vi "FPGA_main_AIchar_v3.vi"() -> ()   [LabVIEW 2020]
doc: "AI from AI modules, Mod6, Mod7, Mod8"
uses:
  <vilib>/rvi/Emulation/niFpgaGetClockAttributes.vi
  <vilib>/rvi/Emulation/niFpgaSctlEmulationGetInTimedLoop.vi
  <vilib>/rvi/Emulation/niFpgaEmulationReportErrorSimple.vi
  <vilib>/rvi/eio/common/nirviEmuTemplateMethod_errors.vi
  <vilib>/rvi/Emulation/niFpgaEmulationIsFPGAContextNoSignature.vi
  <vilib>/rvi/errors/niFpgaSetErrorForExecOnDevCompSimple.vi
  <vilib>/rvi/eio/common/nirviEmuReportErrorAndStop.vi
  <vilib>/rvi/DataTransferAndStorage/Container/Common/niFpgaContainerGetUniqueNameForEmu.vi
  <vilib>/rvi/FIFO/Fifo_Resource/nirvififoEmulationSetSize.vi
  <vilib>/rvi/FIFO/Fifo_Resource/nirviFifoEmulationQueueMgr.vi
  <instcachedir>/0/nirviFifoEmulationQueueMgr_E5CAEC123FF24DC58D834DCA3CDAA9B5.lvgen/nirviFifoEmulationQueueMgr_E5CAEC123FF24DC58D834DCA3CDAA9B5_001.vi
  <vilib>/rvi/FIFO/Fifo_Resource/nirvififoEmulationDetermineInputValidOut.vi
  <vilib>/rvi/FIFO/Fifo_Resource/nirvififoEmulationCreateLock.vi
  <vilib>/rvi/Emulation/niFpgaProcessEmulError.vi
  <vilib>/rvi/FIFO/Fifo_Resource/nirvififoEmulationObtainLock.vi
  <vilib>/rvi/FIFO/Fifo_Resource/nirvififoEmulationReleaseLock.vi
  <vilib>/rvi/occurrence/nirviWaitOnOccurrenceBase.vi
  <vilib>/rvi/errors/nirviReportUnexpectedCaseInternalError.vi
  <vilib>/rvi/errors/nirviReportUnexpectedCaseInternalError (U32).vi
  <vilib>/rvi/Emulation/niFpgaCriticalErrorInLSC.vi
  <vilib>/Utility/error.llb/Clear Errors.vi
  Components/PositionMeas/MovingAverage/256ptMovingAvg.vi
  Components/PositionMeas/MovingAverage/64ptMovingAvg.vi
  <vilib>/rvi/DataTransferAndStorage/Container/Common/niFpgaContainerSetEmuInfo.vi
  <vilib>/eio/EIONode/EIONode.xnode
  <vilib>/rvi/DataTransferAndStorage/Container/XNode/niFpgaContainer.xnode
  <vilib>/rvi/FIFO/Fifo_Resource/nirvififoEmulationWrite.vi
  <vilib>/rvi/FIFO/Fifo_Resource/nirvififoEmulationRead.vi
  <vilib>/rvi/LocalResourceManager/LocalResourceManager.xnode
  Components/PositionMeas/MovingAverage/MovingAvg.lvlib
panel:
  out "AI LS Loop time [us] 2":u8
  out "FPGA AI LS FIFO\nOverflow? 2":bool
  out "AI LS filter Loop time [us] 2":u8
  out "Mod6 (NI 9222) AI":fxp<+/-,25,5>[](array[numeric])
  out "AI LS filter Loop time [us]":u8
  out "Mod7 (NI 9222) AI":fxp<+/-,25,5>[](array[numeric])
  out "AI LS Loop time [us]":u8
  out "FPGA AI LS FIFO\nOverflow?":bool
  out "Mod8 (NI 9222) AI":fxp<+/-,25,5>[](array[numeric])
  out "AI HS filter Loop time [ticks]":u8
  out "FPGA AI HS FIFO\nOverflow?":bool
  out "AI HS Loop time [ticks]":u8
  # "1 tick = 25 ns"
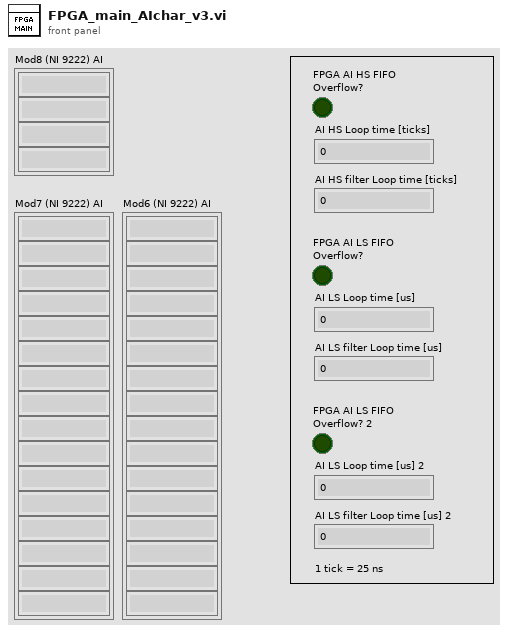
[diagram p1: front panel]
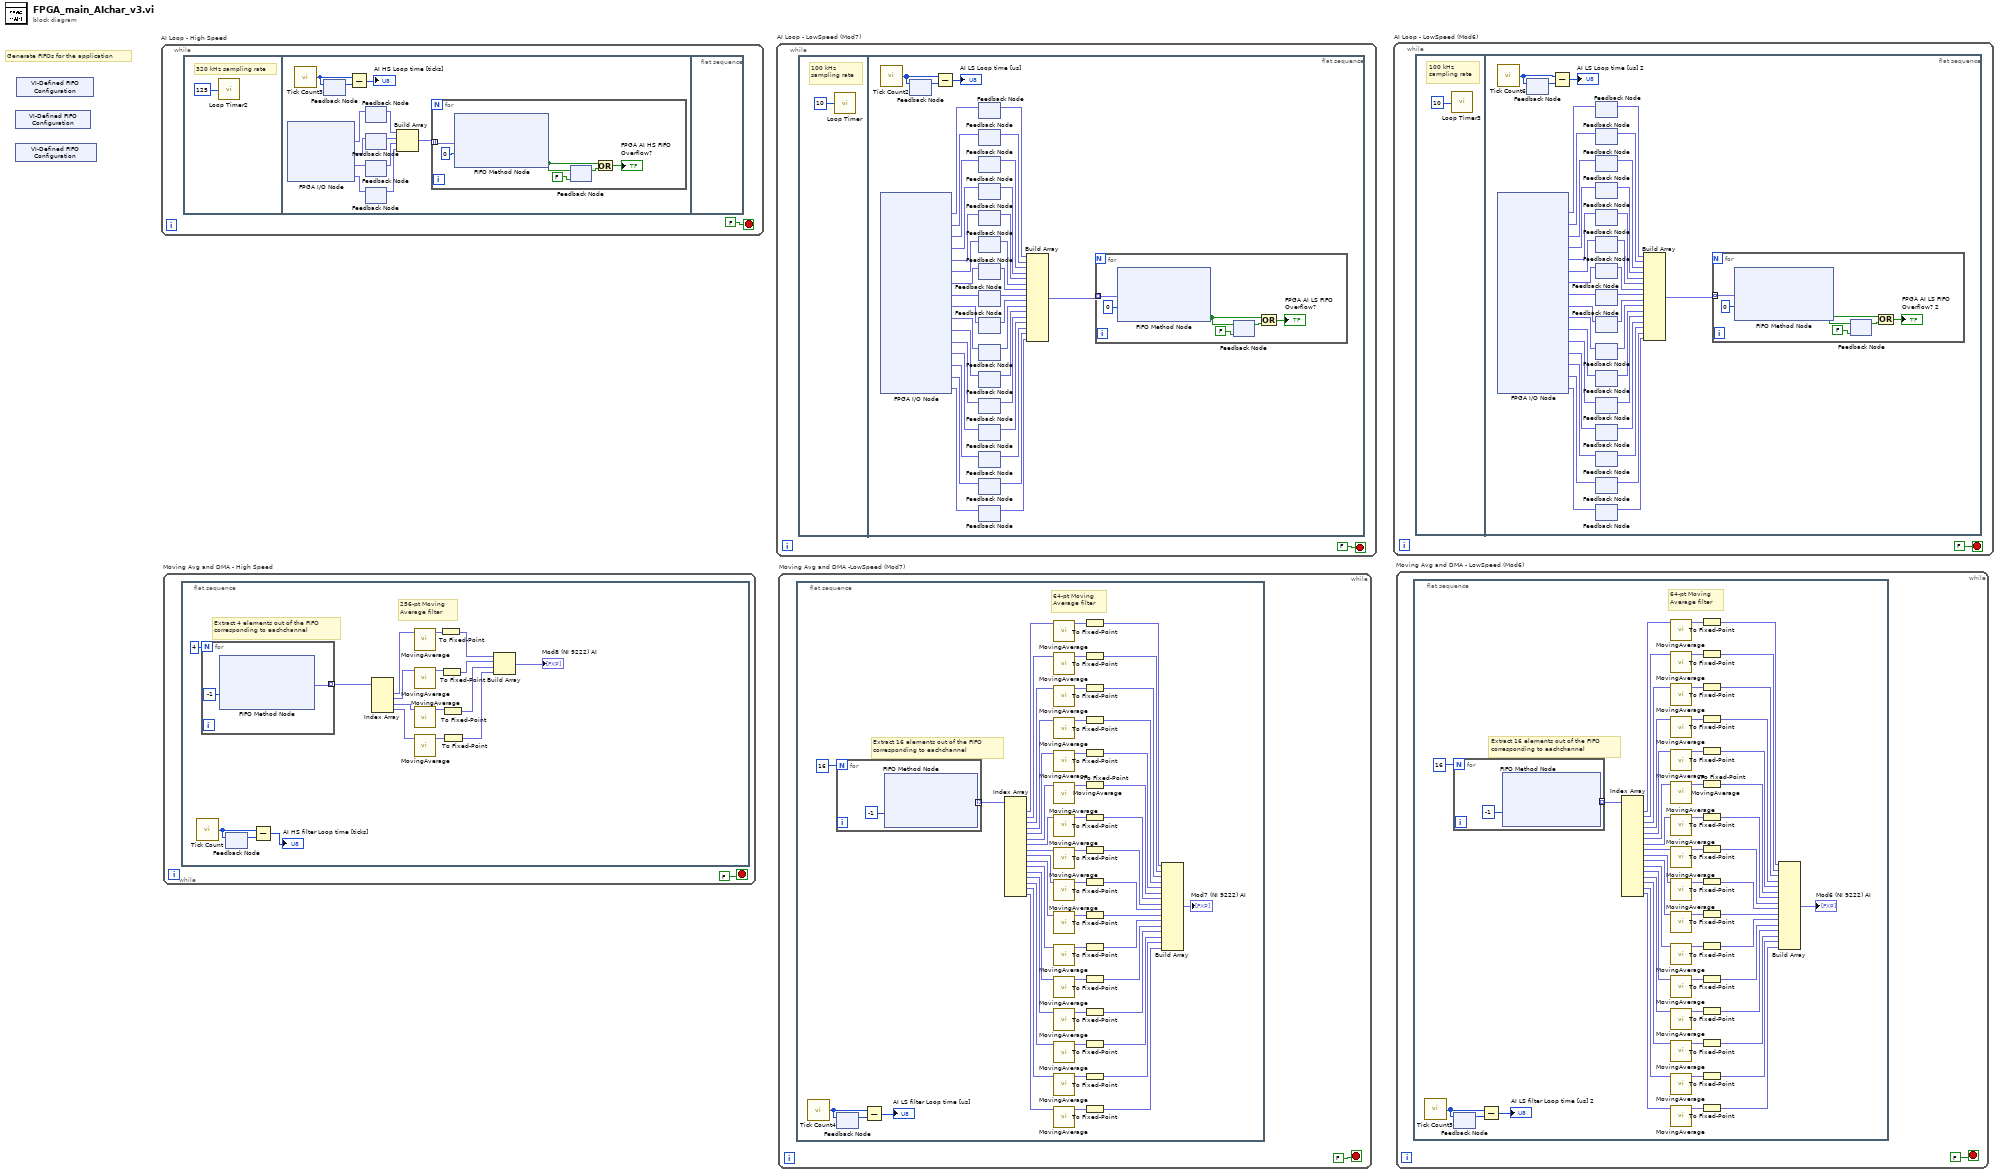
[diagram p0: block diagram]
diagram:
  # "Generate FIFOs for the application"
  n1 = xnode "VI-Defined FIFO Configuration"() -> ()  [unwired: 1 out]
  n2 = xnode "VI-Defined FIFO Configuration"() -> ()  [unwired: 1 out]
  n3 = xnode "VI-Defined FIFO Configuration"() -> ()  [unwired: 1 out]
  n4 = while "AI Loop - High Speed" {
    stop <- FALSE stop-if-true
    n5 = flat-sequence {
      frame #0 {
        # "320 kHz sampling rate"
        n6 = call "Loop Timer2"("Count(Ticks)"=u8 125) -> ()  [unwired: 1 out]
      }
      frame #1 {
        n7 = xnode "FPGA I/O Node"() -> ("Mod8/AI0"=w9:fxp<+/-,24,5>, "Mod8/AI1"=w8:fxp<+/-,24,5>, "Mod8/AI2"=w7:fxp<+/-,24,5>, "Mod8/AI3"=w6:fxp<+/-,24,5>)  [unwired: 4 in, 4 out]
        n8 = call "Tick Count3"() -> ("Tick Count(Ticks)"=w14:u8)
        n9 = feedback #1() -> (w13:u8)  [unwired: 1 in]
        n10 = feedback-in #1(w14) -> ()
        n11 = Subtract(x=w14, y=w13) -> (x-y=→"AI HS Loop time [ticks]":u8)
        n12 = feedback-in #2(w9) -> ()
        n13 = feedback #2() -> (w10:fxp<+/-,24,5>)  [unwired: 1 in]
        n14 = feedback #3() -> (w5:fxp<+/-,24,5>)  [unwired: 1 in]
        n15 = feedback-in #3(w8) -> ()
        n16 = feedback #4() -> (w4:fxp<+/-,24,5>)  [unwired: 1 in]
        n17 = feedback-in #4(w7) -> ()
        n18 = feedback #5() -> (w3:fxp<+/-,24,5>)  [unwired: 1 in]
        n19 = feedback-in #5(w6) -> ()
        n20 = Build Array(w10, w5, w4, w3) -> (w11:fxp<+/-,24,5>[])
        n21 = for {
          tunnel: w11 -> [w19] mode=indexing
          n22 = xnode ("FIFO Method Node")("Element"=w19, "Timeout"=0) -> ("Timed Out?"=w16:bool)  [unwired: 1 in, 1 out]
          n23 = feedback-in #6(w16) -> ()
          n24 = feedback #6(FALSE ("Timed Out?")) -> (w17:bool)
          n25 = Or(x=w16, y=w17) -> (x .or. y?=→"FPGA AI HS FIFO\nOverflow?":bool)
        }
      }
      frame #2 {
      }
    }
  }
  n26 = while "Moving Avg and DMA - High Speed" {
    stop <- FALSE stop-if-true
    n27 = flat-sequence {
      frame #0 {
        # "256-pt Moving \nAverage filter"
        # "Extract 4 elements out of the FIFO \ncorresponding to eachchannel"
        n28 = call "Tick Count"() -> ("Tick Count(Ticks)"=w38:u8)
        n29 = for {
          N: 4 -> [_]
          tunnel: [w40] -> w35 mode=indexing
          n30 = xnode ("FIFO Method Node")("Timeout"=-1) -> ("Element"=w40:fxp<+/-,24,5>)  [unwired: 1 in, 2 out]
        }
        n31 = feedback #7() -> (w37:u8)  [unwired: 1 in]
        n32 = feedback-in #7(w38) -> ()
        n33 = Subtract(x=w38, y=w37) -> (x-y=→"AI HS filter Loop time [ticks]":u8)
        n34 = Index Array(array=w35) -> (element #1=w34:fxp<+/-,24,5>, element #2=w33:fxp<+/-,24,5>, element #3=w31:fxp<+/-,24,5>, element #4=w32:fxp<+/-,24,5>)  [unwired: 4 in]
        n35 = call-poly "MovingAverage.vi"("Raw input"=w34) -> ("Output"=w30:fxp<+/-,28,5>)  [unwired: 10 in]
        n36 = call-poly "MovingAverage.vi"("Raw input"=w33) -> ("Output"=w28:fxp<+/-,28,5>)  [unwired: 10 in]
        n37 = call-poly "MovingAverage.vi"("Raw input"=w31) -> ("Output"=w27:fxp<+/-,28,5>)  [unwired: 10 in]
        n38 = call-poly "MovingAverage.vi"("Raw input"=w32) -> ("Output"=w24:fxp<+/-,28,5>)  [unwired: 10 in]
        n39 = To Fixed-Point(number=w30) -> (fixed-point=w29:fxp<+/-,25,5>)  [unwired: 1 in]
        n40 = To Fixed-Point(number=w28) -> (fixed-point=w26:fxp<+/-,25,5>)  [unwired: 1 in]
        n41 = To Fixed-Point(number=w27) -> (fixed-point=w25:fxp<+/-,25,5>)  [unwired: 1 in]
        n42 = To Fixed-Point(number=w24) -> (fixed-point=w23:fxp<+/-,25,5>)  [unwired: 1 in]
        n43 = Build Array(w29, w26, w25, w23) -> (→"Mod8 (NI 9222) AI":fxp<+/-,25,5>[])
      }
    }
  }
  n44 = while "AI Loop - LowSpeed (Mod7)" {
    stop <- FALSE stop-if-true
    n45 = flat-sequence {
      frame #0 {
        # "100 kHz \nsampling rate"
        n46 = call "Loop Timer"("Count(uSec)"=u8 10 ("Count(Ticks)")) -> ()  [unwired: 1 out]
      }
      frame #1 {
        n47 = call "Tick Count2"() -> ("Tick Count(uSec)"=w79:u8)
        n48 = xnode "FPGA I/O Node"() -> ("Mod7/AI0"=w75:fxp<+/-,24,5>, "Mod7/AI1"=w74:fxp<+/-,24,5>, "Mod7/AI2"=w73:fxp<+/-,24,5>, "Mod7/AI3"=w72:fxp<+/-,24,5>, "Mod7/AI4"=w71:fxp<+/-,24,5>, "Mod7/AI5"=w70:fxp<+/-,24,5>, "Mod7/AI6"=w69:fxp<+/-,24,5>, "Mod7/AI7"=w68:fxp<+/-,24,5>, "Mod7/AI8"=w67:fxp<+/-,24,5>, "Mod7/AI9"=w66:fxp<+/-,24,5>, "Mod7/AI10"=w65:fxp<+/-,24,5>, "Mod7/AI11"=w64:fxp<+/-,24,5>, "Mod7/AI12"=w63:fxp<+/-,24,5>, "Mod7/AI13"=w62:fxp<+/-,24,5>, "Mod7/AI14"=w61:fxp<+/-,24,5>, "Mod7/AI15"=w60:fxp<+/-,24,5>)  [unwired: 16 in, 16 out]
        n49 = feedback #8() -> (w78:u8)  [unwired: 1 in]
        n50 = feedback-in #8(w79) -> ()
        n51 = Subtract(x=w79, y=w78) -> (x-y=→"AI LS Loop time [us]":u8)
        n52 = feedback #9() -> (w59:fxp<+/-,24,5>)  [unwired: 1 in]
        n53 = feedback-in #9(w75) -> ()
        n54 = feedback #10() -> (w58:fxp<+/-,24,5>)  [unwired: 1 in]
        n55 = feedback-in #10(w74) -> ()
        n56 = feedback #11() -> (w57:fxp<+/-,24,5>)  [unwired: 1 in]
        n57 = feedback-in #11(w73) -> ()
        n58 = feedback #12() -> (w56:fxp<+/-,24,5>)  [unwired: 1 in]
        n59 = feedback-in #12(w72) -> ()
        n60 = feedback #13() -> (w55:fxp<+/-,24,5>)  [unwired: 1 in]
        n61 = feedback-in #13(w71) -> ()
        n62 = feedback #14() -> (w54:fxp<+/-,24,5>)  [unwired: 1 in]
        n63 = feedback-in #14(w70) -> ()
        n64 = feedback #15() -> (w53:fxp<+/-,24,5>)  [unwired: 1 in]
        n65 = feedback-in #15(w69) -> ()
        n66 = feedback #16() -> (w52:fxp<+/-,24,5>)  [unwired: 1 in]
        n67 = feedback-in #16(w68) -> ()
        n68 = feedback #17() -> (w51:fxp<+/-,24,5>)  [unwired: 1 in]
        n69 = feedback-in #17(w67) -> ()
        n70 = feedback #18() -> (w50:fxp<+/-,24,5>)  [unwired: 1 in]
        n71 = feedback-in #18(w66) -> ()
        n72 = feedback #19() -> (w49:fxp<+/-,24,5>)  [unwired: 1 in]
        n73 = feedback-in #19(w65) -> ()
        n74 = feedback #20() -> (w48:fxp<+/-,24,5>)  [unwired: 1 in]
        n75 = feedback-in #20(w64) -> ()
        n76 = feedback #21() -> (w47:fxp<+/-,24,5>)  [unwired: 1 in]
        n77 = feedback-in #21(w63) -> ()
        n78 = feedback #22() -> (w46:fxp<+/-,24,5>)  [unwired: 1 in]
        n79 = feedback-in #22(w62) -> ()
        n80 = feedback #23() -> (w45:fxp<+/-,24,5>)  [unwired: 1 in]
        n81 = feedback-in #23(w61) -> ()
        n82 = feedback #24() -> (w44:fxp<+/-,24,5>)  [unwired: 1 in]
        n83 = feedback-in #24(w60) -> ()
        n84 = Build Array(w59, w58, w57, w56, w55, w54, w53, w52, w51, w50, w49, w48, w47, w46, w45, w44) -> (w76:fxp<+/-,24,5>[])
        n85 = for {
          tunnel: w76 -> [w80] mode=indexing
          n86 = xnode ("FIFO Method Node")("Element"=w80, "Timeout"=0) -> ("Timed Out?"=w82:bool)  [unwired: 1 in, 1 out]
          n87 = feedback-in #25(w82) -> ()
          n88 = feedback #25(FALSE ("Timed Out?")) -> (w83:bool)
          n89 = Or(x=w82, y=w83) -> (x .or. y?=→"FPGA AI LS FIFO\nOverflow?":bool)
        }
      }
    }
  }
  n90 = while "Moving Avg and DMA -LowSpeed (Mod7)" {
    stop <- FALSE stop-if-true
    n91 = flat-sequence {
      frame #0 {
        # "64-pt Moving \nAverage filter"
        # "Extract 16 elements out of the FIFO \ncorresponding to eachchannel"
        n92 = call "Tick Count4"() -> ("Tick Count(uSec)"=w139:u8)
        n93 = for {
          N: 16 -> [_]
          tunnel: [w141] -> w136 mode=indexing
          n94 = xnode ("FIFO Method Node")("Timeout"=-1) -> ("Element"=w141:fxp<+/-,24,5>)  [unwired: 1 in, 2 out]
        }
        n95 = feedback #26() -> (w138:u8)  [unwired: 1 in]
        n96 = feedback-in #26(w139) -> ()
        n97 = Subtract(x=w139, y=w138) -> (x-y=→"AI LS filter Loop time [us]":u8)
        n98 = Index Array(array=w136) -> (element #1=w133:fxp<+/-,24,5>, element #2=w132:fxp<+/-,24,5>, element #3=w131:fxp<+/-,24,5>, element #4=w130:fxp<+/-,24,5>, element #5=w129:fxp<+/-,24,5>, element #6=w128:fxp<+/-,24,5>, element #7=w127:fxp<+/-,24,5>, element #8=w126:fxp<+/-,24,5>, element #9=w125:fxp<+/-,24,5>, element #10=w124:fxp<+/-,24,5>, element #11=w123:fxp<+/-,24,5>, element #12=w122:fxp<+/-,24,5>, element #13=w121:fxp<+/-,24,5>, element #14=w120:fxp<+/-,24,5>, element #15=w119:fxp<+/-,24,5>, element #16=w118:fxp<+/-,24,5>)  [unwired: 16 in]
        n99 = call-poly "MovingAverage.vi"("Raw input"=w133) -> ("Output"=w117:fxp<+/-,28,5>)  [unwired: 10 in]
        n100 = call-poly "MovingAverage.vi"("Raw input"=w132) -> ("Output"=w116:fxp<+/-,28,5>)  [unwired: 10 in]
        n101 = call-poly "MovingAverage.vi"("Raw input"=w131) -> ("Output"=w115:fxp<+/-,28,5>)  [unwired: 10 in]
        n102 = call-poly "MovingAverage.vi"("Raw input"=w130) -> ("Output"=w114:fxp<+/-,28,5>)  [unwired: 10 in]
        n103 = call-poly "MovingAverage.vi"("Raw input"=w129) -> ("Output"=w113:fxp<+/-,28,5>)  [unwired: 10 in]
        n104 = call-poly "MovingAverage.vi"("Raw input"=w128) -> ("Output"=w112:fxp<+/-,28,5>)  [unwired: 10 in]
        n105 = call-poly "MovingAverage.vi"("Raw input"=w127) -> ("Output"=w111:fxp<+/-,28,5>)  [unwired: 10 in]
        n106 = call-poly "MovingAverage.vi"("Raw input"=w126) -> ("Output"=w110:fxp<+/-,28,5>)  [unwired: 10 in]
        n107 = call-poly "MovingAverage.vi"("Raw input"=w125) -> ("Output"=w109:fxp<+/-,28,5>)  [unwired: 10 in]
        n108 = call-poly "MovingAverage.vi"("Raw input"=w124) -> ("Output"=w108:fxp<+/-,28,5>)  [unwired: 10 in]
        n109 = call-poly "MovingAverage.vi"("Raw input"=w123) -> ("Output"=w107:fxp<+/-,28,5>)  [unwired: 10 in]
        n110 = call-poly "MovingAverage.vi"("Raw input"=w122) -> ("Output"=w106:fxp<+/-,28,5>)  [unwired: 10 in]
        n111 = call-poly "MovingAverage.vi"("Raw input"=w121) -> ("Output"=w105:fxp<+/-,28,5>)  [unwired: 10 in]
        n112 = call-poly "MovingAverage.vi"("Raw input"=w120) -> ("Output"=w104:fxp<+/-,28,5>)  [unwired: 10 in]
        n113 = call-poly "MovingAverage.vi"("Raw input"=w119) -> ("Output"=w103:fxp<+/-,28,5>)  [unwired: 10 in]
        n114 = call-poly "MovingAverage.vi"("Raw input"=w118) -> ("Output"=w102:fxp<+/-,28,5>)  [unwired: 10 in]
        n115 = To Fixed-Point(number=w117) -> (fixed-point=w135:fxp<+/-,25,5>)  [unwired: 1 in]
        n116 = To Fixed-Point(number=w116) -> (fixed-point=w101:fxp<+/-,25,5>)  [unwired: 1 in]
        n117 = To Fixed-Point(number=w115) -> (fixed-point=w100:fxp<+/-,25,5>)  [unwired: 1 in]
        n118 = To Fixed-Point(number=w114) -> (fixed-point=w99:fxp<+/-,25,5>)  [unwired: 1 in]
        n119 = To Fixed-Point(number=w113) -> (fixed-point=w98:fxp<+/-,25,5>)  [unwired: 1 in]
        n120 = To Fixed-Point(number=w112) -> (fixed-point=w97:fxp<+/-,25,5>)  [unwired: 1 in]
        n121 = To Fixed-Point(number=w111) -> (fixed-point=w96:fxp<+/-,25,5>)  [unwired: 1 in]
        n122 = To Fixed-Point(number=w110) -> (fixed-point=w95:fxp<+/-,25,5>)  [unwired: 1 in]
        n123 = To Fixed-Point(number=w109) -> (fixed-point=w94:fxp<+/-,25,5>)  [unwired: 1 in]
        n124 = To Fixed-Point(number=w108) -> (fixed-point=w93:fxp<+/-,25,5>)  [unwired: 1 in]
        n125 = To Fixed-Point(number=w107) -> (fixed-point=w92:fxp<+/-,25,5>)  [unwired: 1 in]
        n126 = To Fixed-Point(number=w106) -> (fixed-point=w91:fxp<+/-,25,5>)  [unwired: 1 in]
        n127 = To Fixed-Point(number=w105) -> (fixed-point=w90:fxp<+/-,25,5>)  [unwired: 1 in]
        n128 = To Fixed-Point(number=w104) -> (fixed-point=w89:fxp<+/-,25,5>)  [unwired: 1 in]
        n129 = To Fixed-Point(number=w103) -> (fixed-point=w88:fxp<+/-,25,5>)  [unwired: 1 in]
        n130 = To Fixed-Point(number=w102) -> (fixed-point=w87:fxp<+/-,25,5>)  [unwired: 1 in]
        n131 = Build Array(w135, w101, w100, w99, w98, w97, w96, w95, w94, w93, w92, w91, w90, w89, w88, w87) -> (→"Mod7 (NI 9222) AI":fxp<+/-,25,5>[])
      }
    }
  }
  n132 = while "AI Loop - LowSpeed (Mod6)" {
    stop <- FALSE stop-if-true
    n133 = flat-sequence {
      frame #0 {
        # "100 kHz \nsampling rate"
        n134 = call "Loop Timer3"("Count(uSec)"=u8 10 ("Count(Ticks)")) -> ()  [unwired: 1 out]
      }
      frame #1 {
        n135 = call "Tick Count6"() -> ("Tick Count(uSec)"=w180:u8)
        n136 = xnode "FPGA I/O Node"() -> ("Mod6/AI0"=w176:fxp<+/-,24,5>, "Mod6/AI1"=w159:fxp<+/-,24,5>, "Mod6/AI2"=w158:fxp<+/-,24,5>, "Mod6/AI3"=w157:fxp<+/-,24,5>, "Mod6/AI4"=w156:fxp<+/-,24,5>, "Mod6/AI5"=w155:fxp<+/-,24,5>, "Mod6/AI6"=w154:fxp<+/-,24,5>, "Mod6/AI7"=w153:fxp<+/-,24,5>, "Mod6/AI8"=w152:fxp<+/-,24,5>, "Mod6/AI9"=w151:fxp<+/-,24,5>, "Mod6/AI10"=w150:fxp<+/-,24,5>, "Mod6/AI11"=w149:fxp<+/-,24,5>, "Mod6/AI12"=w148:fxp<+/-,24,5>, "Mod6/AI13"=w147:fxp<+/-,24,5>, "Mod6/AI14"=w146:fxp<+/-,24,5>, "Mod6/AI15"=w145:fxp<+/-,24,5>)  [unwired: 16 in, 16 out]
        n137 = feedback #27() -> (w179:u8)  [unwired: 1 in]
        n138 = feedback-in #27(w180) -> ()
        n139 = Subtract(x=w180, y=w179) -> (x-y=→"AI LS Loop time [us] 2":u8)
        n140 = feedback #28() -> (w175:fxp<+/-,24,5>)  [unwired: 1 in]
        n141 = feedback-in #28(w176) -> ()
        n142 = feedback #29() -> (w174:fxp<+/-,24,5>)  [unwired: 1 in]
        n143 = feedback-in #29(w159) -> ()
        n144 = feedback #30() -> (w173:fxp<+/-,24,5>)  [unwired: 1 in]
        n145 = feedback-in #30(w158) -> ()
        n146 = feedback #31() -> (w172:fxp<+/-,24,5>)  [unwired: 1 in]
        n147 = feedback-in #31(w157) -> ()
        n148 = feedback #32() -> (w171:fxp<+/-,24,5>)  [unwired: 1 in]
        n149 = feedback-in #32(w156) -> ()
        n150 = feedback #33() -> (w170:fxp<+/-,24,5>)  [unwired: 1 in]
        n151 = feedback-in #33(w155) -> ()
        n152 = feedback #34() -> (w169:fxp<+/-,24,5>)  [unwired: 1 in]
        n153 = feedback-in #34(w154) -> ()
        n154 = feedback #35() -> (w168:fxp<+/-,24,5>)  [unwired: 1 in]
        n155 = feedback-in #35(w153) -> ()
        n156 = feedback #36() -> (w167:fxp<+/-,24,5>)  [unwired: 1 in]
        n157 = feedback-in #36(w152) -> ()
        n158 = feedback #37() -> (w166:fxp<+/-,24,5>)  [unwired: 1 in]
        n159 = feedback-in #37(w151) -> ()
        n160 = feedback #38() -> (w165:fxp<+/-,24,5>)  [unwired: 1 in]
        n161 = feedback-in #38(w150) -> ()
        n162 = feedback #39() -> (w164:fxp<+/-,24,5>)  [unwired: 1 in]
        n163 = feedback-in #39(w149) -> ()
        n164 = feedback #40() -> (w163:fxp<+/-,24,5>)  [unwired: 1 in]
        n165 = feedback-in #40(w148) -> ()
        n166 = feedback #41() -> (w162:fxp<+/-,24,5>)  [unwired: 1 in]
        n167 = feedback-in #41(w147) -> ()
        n168 = feedback #42() -> (w161:fxp<+/-,24,5>)  [unwired: 1 in]
        n169 = feedback-in #42(w146) -> ()
        n170 = feedback #43() -> (w160:fxp<+/-,24,5>)  [unwired: 1 in]
        n171 = feedback-in #43(w145) -> ()
        n172 = Build Array(w175, w174, w173, w172, w171, w170, w169, w168, w167, w166, w165, w164, w163, w162, w161, w160) -> (w177:fxp<+/-,24,5>[])
        n173 = for {
          tunnel: w177 -> [w181] mode=indexing
          n174 = xnode ("FIFO Method Node")("Element"=w181, "Timeout"=0) -> ("Timed Out?"=w183:bool)  [unwired: 1 in, 1 out]
          n175 = feedback-in #44(w183) -> ()
          n176 = feedback #44(FALSE ("Timed Out?")) -> (w184:bool)
          n177 = Or(x=w183, y=w184) -> (x .or. y?=→"FPGA AI LS FIFO\nOverflow? 2":bool)
        }
      }
    }
  }
  n178 = while "Moving Avg and DMA - LowSpeed (Mod6)" {
    stop <- FALSE stop-if-true
    n179 = flat-sequence {
      frame #0 {
        # "64-pt Moving \nAverage filter"
        # "Extract 16 elements out of the FIFO \ncorresponding to eachchannel"
        n180 = call "Tick Count5"() -> ("Tick Count(uSec)"=w240:u8)
        n181 = for {
          N: 16 -> [_]
          tunnel: [w242] -> w237 mode=indexing
          n182 = xnode ("FIFO Method Node")("Timeout"=-1) -> ("Element"=w242:fxp<+/-,24,5>)  [unwired: 1 in, 2 out]
        }
        n183 = feedback #45() -> (w239:u8)  [unwired: 1 in]
        n184 = feedback-in #45(w240) -> ()
        n185 = Subtract(x=w240, y=w239) -> (x-y=→"AI LS filter Loop time [us] 2":u8)
        n186 = Index Array(array=w237) -> (element #1=w235:fxp<+/-,24,5>, element #2=w234:fxp<+/-,24,5>, element #3=w233:fxp<+/-,24,5>, element #4=w232:fxp<+/-,24,5>, element #5=w231:fxp<+/-,24,5>, element #6=w230:fxp<+/-,24,5>, element #7=w229:fxp<+/-,24,5>, element #8=w228:fxp<+/-,24,5>, element #9=w227:fxp<+/-,24,5>, element #10=w226:fxp<+/-,24,5>, element #11=w225:fxp<+/-,24,5>, element #12=w224:fxp<+/-,24,5>, element #13=w223:fxp<+/-,24,5>, element #14=w222:fxp<+/-,24,5>, element #15=w221:fxp<+/-,24,5>, element #16=w220:fxp<+/-,24,5>)  [unwired: 16 in]
        n187 = call-poly "MovingAverage.vi"("Raw input"=w235) -> ("Output"=w219:fxp<+/-,28,5>)  [unwired: 10 in]
        n188 = call-poly "MovingAverage.vi"("Raw input"=w234) -> ("Output"=w218:fxp<+/-,28,5>)  [unwired: 10 in]
        n189 = call-poly "MovingAverage.vi"("Raw input"=w233) -> ("Output"=w217:fxp<+/-,28,5>)  [unwired: 10 in]
        n190 = call-poly "MovingAverage.vi"("Raw input"=w232) -> ("Output"=w216:fxp<+/-,28,5>)  [unwired: 10 in]
        n191 = call-poly "MovingAverage.vi"("Raw input"=w231) -> ("Output"=w215:fxp<+/-,28,5>)  [unwired: 10 in]
        n192 = call-poly "MovingAverage.vi"("Raw input"=w230) -> ("Output"=w214:fxp<+/-,28,5>)  [unwired: 10 in]
        n193 = call-poly "MovingAverage.vi"("Raw input"=w229) -> ("Output"=w213:fxp<+/-,28,5>)  [unwired: 10 in]
        n194 = call-poly "MovingAverage.vi"("Raw input"=w228) -> ("Output"=w212:fxp<+/-,28,5>)  [unwired: 10 in]
        n195 = call-poly "MovingAverage.vi"("Raw input"=w227) -> ("Output"=w211:fxp<+/-,28,5>)  [unwired: 10 in]
        n196 = call-poly "MovingAverage.vi"("Raw input"=w226) -> ("Output"=w210:fxp<+/-,28,5>)  [unwired: 10 in]
        n197 = call-poly "MovingAverage.vi"("Raw input"=w225) -> ("Output"=w209:fxp<+/-,28,5>)  [unwired: 10 in]
        n198 = call-poly "MovingAverage.vi"("Raw input"=w224) -> ("Output"=w208:fxp<+/-,28,5>)  [unwired: 10 in]
        n199 = call-poly "MovingAverage.vi"("Raw input"=w223) -> ("Output"=w207:fxp<+/-,28,5>)  [unwired: 10 in]
        n200 = call-poly "MovingAverage.vi"("Raw input"=w222) -> ("Output"=w206:fxp<+/-,28,5>)  [unwired: 10 in]
        n201 = call-poly "MovingAverage.vi"("Raw input"=w221) -> ("Output"=w205:fxp<+/-,28,5>)  [unwired: 10 in]
        n202 = call-poly "MovingAverage.vi"("Raw input"=w220) -> ("Output"=w204:fxp<+/-,28,5>)  [unwired: 10 in]
        n203 = To Fixed-Point(number=w219) -> (fixed-point=w236:fxp<+/-,25,5>)  [unwired: 1 in]
        n204 = To Fixed-Point(number=w218) -> (fixed-point=w203:fxp<+/-,25,5>)  [unwired: 1 in]
        n205 = To Fixed-Point(number=w217) -> (fixed-point=w202:fxp<+/-,25,5>)  [unwired: 1 in]
        n206 = To Fixed-Point(number=w216) -> (fixed-point=w201:fxp<+/-,25,5>)  [unwired: 1 in]
        n207 = To Fixed-Point(number=w215) -> (fixed-point=w200:fxp<+/-,25,5>)  [unwired: 1 in]
        n208 = To Fixed-Point(number=w214) -> (fixed-point=w199:fxp<+/-,25,5>)  [unwired: 1 in]
        n209 = To Fixed-Point(number=w213) -> (fixed-point=w198:fxp<+/-,25,5>)  [unwired: 1 in]
        n210 = To Fixed-Point(number=w212) -> (fixed-point=w197:fxp<+/-,25,5>)  [unwired: 1 in]
        n211 = To Fixed-Point(number=w211) -> (fixed-point=w196:fxp<+/-,25,5>)  [unwired: 1 in]
        n212 = To Fixed-Point(number=w210) -> (fixed-point=w195:fxp<+/-,25,5>)  [unwired: 1 in]
        n213 = To Fixed-Point(number=w209) -> (fixed-point=w194:fxp<+/-,25,5>)  [unwired: 1 in]
        n214 = To Fixed-Point(number=w208) -> (fixed-point=w193:fxp<+/-,25,5>)  [unwired: 1 in]
        n215 = To Fixed-Point(number=w207) -> (fixed-point=w192:fxp<+/-,25,5>)  [unwired: 1 in]
        n216 = To Fixed-Point(number=w206) -> (fixed-point=w191:fxp<+/-,25,5>)  [unwired: 1 in]
        n217 = To Fixed-Point(number=w205) -> (fixed-point=w190:fxp<+/-,25,5>)  [unwired: 1 in]
        n218 = To Fixed-Point(number=w204) -> (fixed-point=w189:fxp<+/-,25,5>)  [unwired: 1 in]
        n219 = Build Array(w236, w203, w202, w201, w200, w199, w198, w197, w196, w195, w194, w193, w192, w191, w190, w189) -> (→"Mod6 (NI 9222) AI":fxp<+/-,25,5>[])
      }
    }
  }
